vi "Monitoring Data.vi"() -> ()   [LabVIEW 2011, in "Controller Global Variables.lvlib"]
uses:
  Controller Global Variables.lvlib
  Types Definitions/Type Monitoring Data.ctl
  Types Definitions/Type Diagnostics Data.ctl
  Types Definitions/Type CPU Loads Array.ctl
  Types Definitions/Type CPU Loads.ctl
  Type Definitions.lvlib
panel:
  in  "Monitoring Data":T1 {"Diagnostics Data"."CPU Loads Array"."ISR (%)" format="%#.2f"; "Diagnostics Data"."CPU Loads Array"."Idle (%)" format="%#.2f"; "Diagnostics Data"."CPU Loads Array"."Background (%)" format="%#.2f"; "Diagnostics Data"."CPU Loads Array"."Normal (%)" format="%#.2f"; "Diagnostics Data"."CPU Loads Array"."Above Normal (%)" format="%#.2f"; "Diagnostics Data"."CPU Loads Array"."High (%)" format="%#.2f"; "Diagnostics Data"."CPU Loads Array"."Timed Structures (%)" format="%#.2f"; "Diagnostics Data"."CPU Loads Array"."Time Critical (%)" format="%#.2f"; "Diagnostics Data"."CPU Loads Array"."Total (%)" format="%#.2f"}
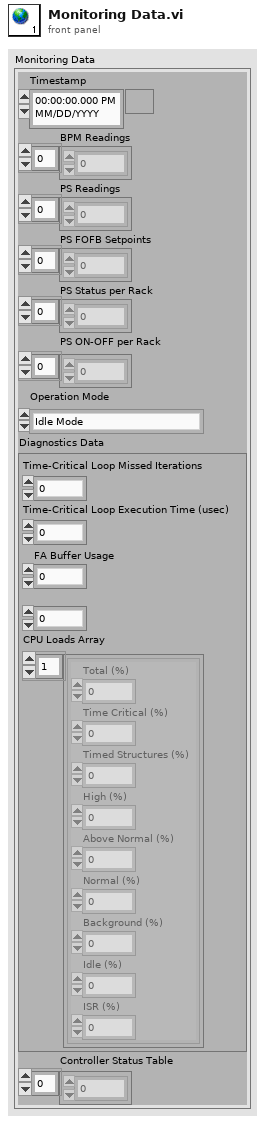
[diagram p1: front panel]
types:
  T1 = typedef "Type Definitions.lvlib/Type Monitoring Data.ctl" = cluster{"Timestamp":timestamp, "BPM Readings":dbl[], "PS Readings":dbl[], "PS FOFB Setpoints":dbl[], "PS Status per Rack":u8[], "PS ON-OFF per Rack":u8[], "Operation Mode":enum16{"Idle Mode", "Error Mode", "Manual Mode", "FOFB Mode", "RMM Mode"}, "Diagnostics Data":T2, "Controller Status Table":i32[]}
  T2 = typedef "Type Definitions.lvlib/Type Diagnostics Data.ctl" = cluster{"Time-Critical Loop Missed Iterations":u32, "Time-Critical Loop Execution Time (usec)":u32, "FA Buffer Usage":u32, "Available Memory (bytes)":u32, "CPU Loads Array":T3}
  T3 = typedef "Type Definitions.lvlib/Type CPU Loads Array.ctl" = T4[]
  T4 = typedef "Type Definitions.lvlib/Type CPU Loads.ctl" = cluster{"Total (%)":dbl, "Time Critical (%)":dbl, "Timed Structures (%)":dbl, "High (%)":dbl, "Above Normal (%)":dbl, "Normal (%)":dbl, "Background (%)":dbl, "Idle (%)":dbl, "ISR (%)":dbl}
diagram:
